vi "users parse GET parameters.vi"(8 "error in (no error)":errorcluster, 10 "Current User (none)":T1, 11 "GET (empty)":T2) -> (0 "error out":errorcluster, 2 "Parameter":string, 3 "Command":string)   [LabVIEW 2011]
uses:
  Addons/internet/utils/keyedarr.llb/Keyed Array.ctl
  server/database/Users/User Record.ctl
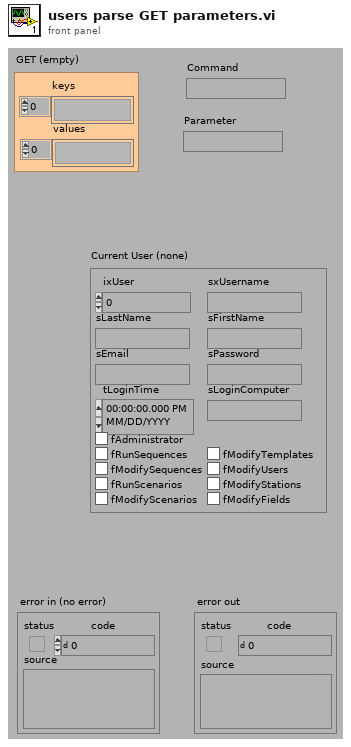
[diagram p1: front panel]
types:
  T1 = typedef "User Record.ctl" = cluster{"ixUser":i32, "sxUsername":string, "sLastName":string, "sFirstName":string, "sEmail":string, "sPassword":string, "tLoginTime":timestamp, "sLoginComputer":string, "fAdministrator":bool, "fRunSequences":bool, "fModifySequences":bool, "fRunScenarios":bool, "fModifyScenarios":bool, "fModifyTemplates":bool, "fModifyUsers":bool, "fModifyStations":bool, "fModifyFields":bool}
  T2 = typedef "Keyed Array.ctl" = cluster{"keys":string[], "values":string[]}
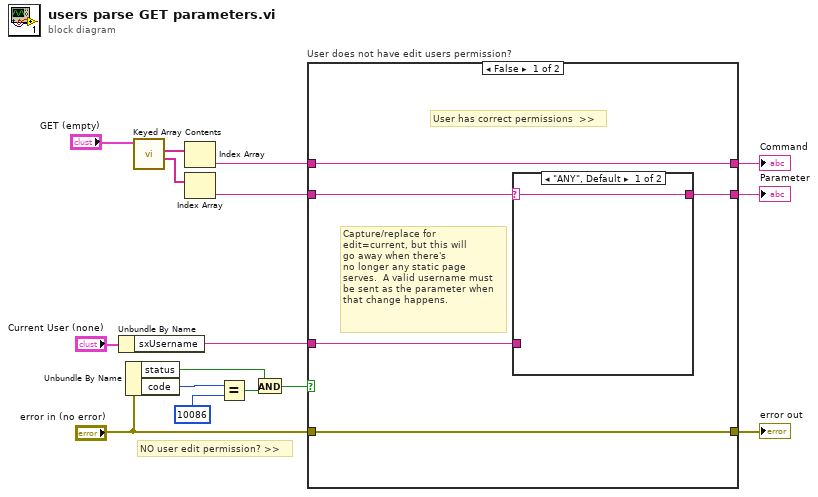
[diagram p0: block diagram]
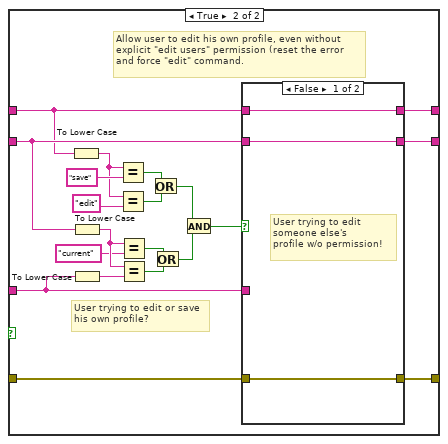
[diagram p3: hidden frame]
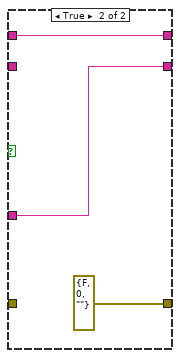
[diagram p4: hidden frame]
diagram:
  # "NO user edit permission? >>"
  n1 = Unbundle By Name("Current User (none)") -> ("sxUsername"=w12:string)
  n2 = Unbundle By Name("error in (no error)") -> ("status"=w8:bool, "code"=w10:i32)
  n3 = call "Keyed Array Contents.vi"("array in"="GET (empty)") -> ("values"=w15:string[], "keys"=w16:string[])  [unwired: 2 in, 3 out]
  n4 = Index Array(array=w16) -> (element=w5:string)  [unwired: 1 in]
  n5 = Index Array(array=w15) -> (element=w11:string)  [unwired: 1 in]
  n6 = Equal?(x=w10, y=10086) -> (x = y?=w7:bool)
  n7 = And(x=w8, y=w7) -> (x .and. y?=w6:bool)
  n8 = case "User does not have edit users permission?" shown="False" w6 {
    tunnel: w12 -> [w18 w24]
    tunnel: w11 -> [w19 w42]
    tunnel: w5 -> [w21 w34]
    tunnel: [w21 w43] -> w4
    tunnel: [w17 w41] -> w3
    tunnel: "error in (no error)" -> [w20 w40]
    tunnel: [w20 w39] -> w1
    frame False {
      # "Capture/replace for \nedit=current, but this will\ngo away when there's\nno longer any static page\nserves.  A valid username must\nbe sent as the parameter when\nthat change happens."
      # "User has correct permissions  >>"
      n9 = case shown="\"ANY\", Default" w19 {
        selector: w19 -> [w22 _]
        tunnel: w18 -> [_ w23]
        tunnel: [w22 w23] -> w17
        frame "ANY", Default {
        }
        frame "current" {
        }
      }
    }
    frame True {
      # "User trying to edit or save\nhis own profile?"
      # "Allow user to edit his own profile, even without\nexplicit \"edit users\" permission (reset the error\nand force \"edit\" command."
      n10 = To Lower Case(string=w34) -> (all lower case string=w32:string)
      n11 = To Lower Case(string=w42) -> (all lower case string=w37:string)
      n12 = To Lower Case(string=w24) -> (all lower case string=w38:string)
      n13 = Equal?(x=w32, y="save") -> (x = y?=w33:bool)
      n14 = Equal?(x=w32, y="edit") -> (x = y?=w30:bool)
      n15 = Equal?(x=w37, y="current") -> (x = y?=w29:bool)
      n16 = Equal?(x=w37, y=w38) -> (x = y?=w28:bool)
      n17 = Or(x=w33, y=w30) -> (x .or. y?=w26:bool)
      n18 = Or(x=w29, y=w28) -> (x .or. y?=w27:bool)
      n19 = And(x=w26, y=w27) -> (x .and. y?=w25:bool)
      n20 = case shown="False" w25 {
        tunnel: w34 -> [w46 w47]
        tunnel: [w46 w47] -> w43
        tunnel: w42 -> [w45 _]
        tunnel: [w45 w48] -> w41
        tunnel: w40 -> [w44 _]
        tunnel: [w44 errorcluster {"status"=FALSE, "code"=0, "source"=""} ("error in (no error)")] -> w39
        tunnel: w24 -> [_ w48]
        frame False {
          # "User trying to edit\nsomeone else's\nprofile w/o permission!"
        }
        frame True {
        }
      }
    }
  }
  "error out" <- w1
  "Command" <- w4
  "Parameter" <- w3
